vi "Dia 3 - Música.vi"() -> ()   [LabVIEW 2017]
panel:
  in  "base tiempo(s)":dbl=0.1
  in  "Duracion_notas: 1:semicorchea":u8[](array[numeric])=[6, 6, 1, 1, 4, 4, 1, 1, 12, 12, 6, 6, 1, 1, 4, 6, 1, 1, 10, 8, 6, 6, 1, 1, 4, 4, 1, 1, 12, 12, 6, 6, 2, 2, 2, 2, 12, 12]
  in  "Notas":dbl[](array[numeric])=[10.0, 3.0, 6.0, 8.0, 10.0, 3.0, 6.0, 8.0, 5.0, 0.0, 8.0, 1.0, 6.0, 5.0, 8.0, 1.0, 6.0, 5.0, 3.0, 0.0, 10.0, 3.0, 6.0, 8.0, 10.0, 3.0, 6.0, 8.0, 5.0, 5.0, 8.0, 1.0, 5.0, 6.0, 5.0, 1.0, 3.0, 3.0]
  # "0: Silenci  1:Do       2:Do#    3:Re      4:Re#      5:Mi        6:Fa       7:Fa#     8:Sol      9:Sol#    10:La      11:La#    12:Si\n     f=0"
  # "0: Silenci  1:Do 2:Do# 3:Re 4:Re# 5:Mi 6:Fa 7:Fa# 8:Sol 9:Sol# 10:La 11:La# 12:Si"
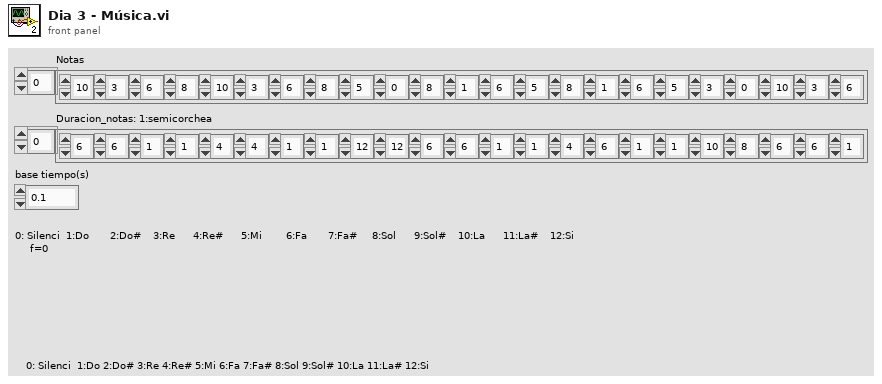
[diagram p1: front panel]
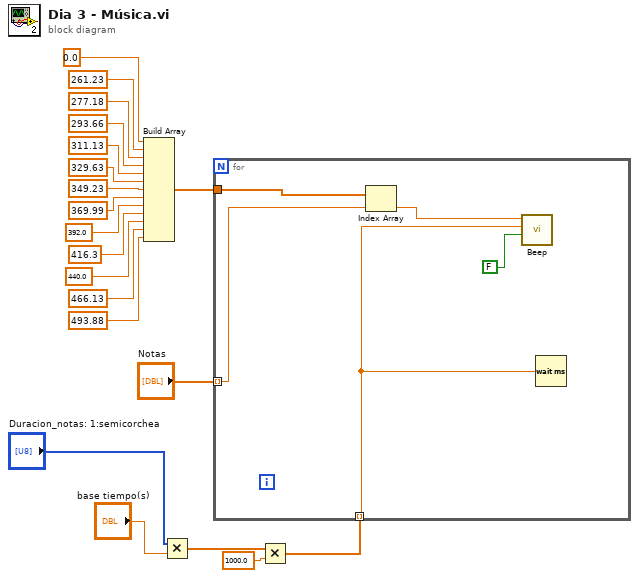
[diagram p0: block diagram]
diagram:
  n1 = Build Array(0.0, 261.23, 277.18, 293.66, 311.13, 329.63, 349.23, 369.99, 392.0, 416.3, 440.0, 466.13, 493.88) -> (w7:dbl[])
  n2 = Multiply(x="Duracion_notas: 1:semicorchea", y="base tiempo(s)") -> (x*y=w5:dbl[])
  n3 = Multiply(x=w5, y=1000.0) -> (x*y=w1:dbl[])
  n4 = for {
    tunnel: w7 -> [w25]
    tunnel: "Notas" -> [w21] mode=indexing
    tunnel: w1 -> [w23] mode=indexing
    n5 = Index Array(array=w25, index=w21) -> (element=w24:dbl)
    n6 = call <vilib>:"Beep.vi"("use system alert? (T)"=FALSE, "duration (msec)"=w23, "frequency (Hz)"=w24) -> ()  [unwired: 9 in]
    n7 = Wait (ms)(milliseconds to wait=w23) -> ()  [unwired: 1 out]
  }
